vi "Class.SaveCtrls.InitLoadRestore.vi"(6 "Ctrl Array":refnum<vi>[](array[refnum]), 8 "error in":errorcluster, 9 "Module Data Dir":path, 10 "Module Name":string, 11 "CtrlStates In":refnum<class "Class.SaveCtrls.lvclass">) -> (0 "error out":errorcluster, 3 "CtrlStates":refnum<class "Class.SaveCtrls.lvclass">)   [LabVIEW 2024, in "EQMF.lvlib" / "Config Utils.lvlib" / "Class.SaveCtrls.lvclass"]
doc: "This VI is intended to be used at the application launch. This VI will input a list of control references, a folder (Module Data Dir) and the Module Name. It will read previously saved control values from the file:\n<Module Data Dir>\\<Module Name>.dat\nThen it will restore each control to its previous value. The list of control references and the file path are saved inside this class and are used by the SaveCtrls.Save.VI (at the application exit). \n\nINPUTS:\n<B>Module Name</B> - The is the name of the SW module that the control are local to. This is used to build the file name where the control values are saved.\n<B>Module Data Dir</B> - The is the path to a folder where application data is stored.\n<B>CtrlArray</B> - The is an array of control references. This is used to obtain the control to read/write its value.\n\nOUTPUTS:\nNone\n\nERRORS: \nAn error will be reported if the file containing the control information cannot be opened."
uses:
  Class.SaveCtrls.lvclass
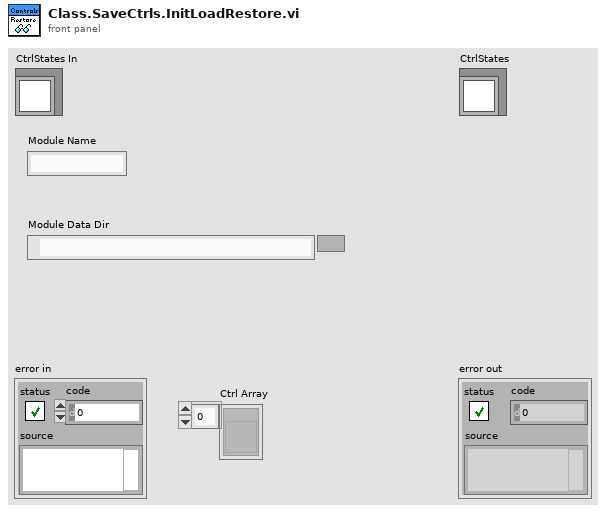
[diagram p1: front panel]
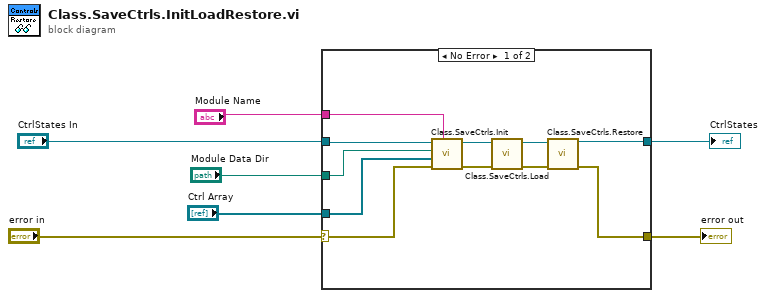
[diagram p0: block diagram]
diagram:
  n1 = case shown="No Error" "error in" {
    selector: "error in" -> [w11 w20]
    tunnel: [w12 w20] -> w6
    tunnel: [w13 w19] -> w4
    tunnel: "CtrlStates In" -> [w14 w19]
    tunnel: "Ctrl Array" -> [w10 _]
    tunnel: "Module Data Dir" -> [w9 _]
    tunnel: "Module Name" -> [w8 _]
    frame No Error {
      n2 = call-dynamic "Class.SaveCtrls.Init.vi"("Module Name"=w8, "error in (no error)"=w11, "Ctrl Array"=w10, "Module Data Dir"=w9, "Save Control States in"=w14) -> ("error out"=w18:errorcluster, "Save Control States out"=w17:refnum<class "Class.SaveCtrls.lvclass">)  [unwired: 5 in]
      n3 = call-dynamic "Class.SaveCtrls.Load.vi"("error in"=w18, "Save Control States in"=w17) -> ("error out"=w16:errorcluster, "Save Control States out"=w15:refnum<class "Class.SaveCtrls.lvclass">)  [unwired: 8 in]
      n4 = call-dynamic "Class.SaveCtrls.Restore.vi"("error in"=w16, "Save Control States in"=w15) -> ("error out"=w12:errorcluster, "Save Control States out"=w13:refnum<class "Class.SaveCtrls.lvclass">)  [unwired: 8 in]
    }
    frame Error {
    }
  }
  "error out" <- w6
  "CtrlStates" <- w4
